vi "MQTT_SubAck_Send.vi"(8 "error in (no error)":errorcluster, 9 "Granted QoS Levels":T2[](array[typedef]), 10 "Message ID":u16=10 format="%x", 11 "SSL_Connection":T1) -> (0 "error out":errorcluster, 2 "Suback Message":u8[](array[numeric]) format="%x", 3 "SSL_Connection":T1)   [LabVIEW 2018, in "AWS_IoT.lvlib"]
uses:
  AWS_IoT.lvlib
  Controls/QoS.ctl
  Controls/SSL_Connection.ctl
  Controls/MessageType.ctl
  Controls/Retain_Flag.ctl
  Controls/DUP_Flag.ctl
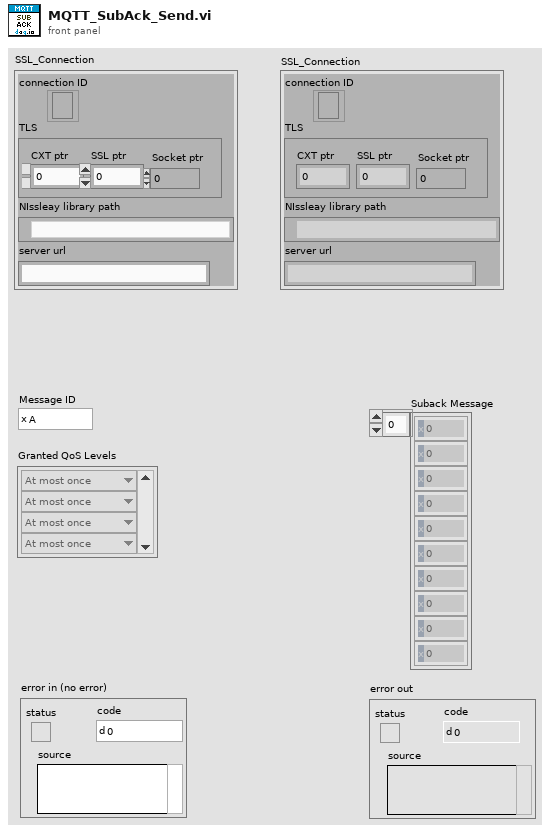
[diagram p1: front panel]
types:
  T1 = typedef "AWS_IoT.lvlib/SSL_Connection.ctl" = cluster{"connection ID":refnum<k5>, "TLS":cluster{"CXT ptr":i32, "SSL ptr":i32, "Socket ptr":i32}, "NIssleay library path":path, "server url":string}
  T2 = typedef "AWS_IoT.lvlib/QoS.ctl" = enum8{"At most once", "At least once", "Exactly once", "Reserved"}
  T3 = typedef "AWS_IoT.lvlib/DUP_Flag.ctl" = bool
  T4 = typedef "AWS_IoT.lvlib/Retain_Flag.ctl" = bool
  T5 = typedef "AWS_IoT.lvlib/MessageType.ctl" = enum32{"Reserved", "CONNECT", "CONNACK", "PUBLISH", "PUBACK", "PUBREC", "PUBREL", "PUBCOMP", "SUBSCRIBE", "SUBACK", "UNSUBSCRIBE", "UNSUBACK", "PINGREQ", "PINGRESP", "DISCONNECT", "Reserved2"}
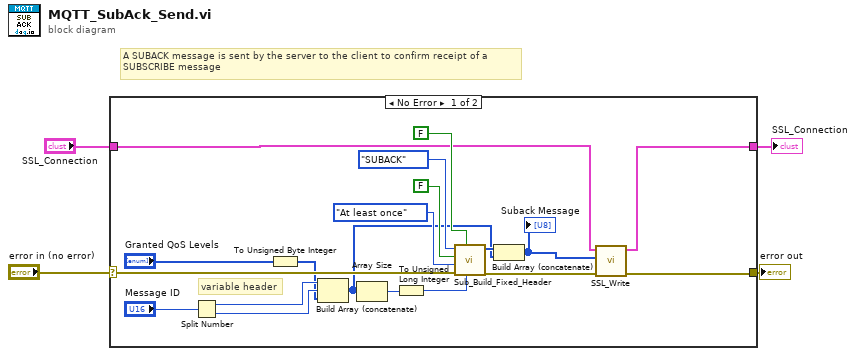
[diagram p0: block diagram]
diagram:
  # "A SUBACK message is sent by the server to the client to confirm receipt of a\nSUBSCRIBE message"
  n1 = case shown="No Error" "error in (no error)" {
    selector: "error in (no error)" -> [w15 w25]
    tunnel: [w9 w25] -> w3
    tunnel: "SSL_Connection" -> [w6 w24]
    tunnel: [w5 w24] -> w1
    frame No Error {
      # "variable header"
      n2 = Split Number(x="Message ID") -> (hi(x)=w21:u8, lo(x)=w20:u8)
      n3 = To Unsigned Byte Integer(number="Granted QoS Levels") -> (unsigned 8bit integer=w10:u8[])
      n4 = Build Array (concatenate)(w21, w20, w10) -> (w14:u8[])
      n5 = Array Size(array=w14) -> (size(s)=w13:i32)
      n6 = To Unsigned Long Integer(number=w13) -> (unsigned 32bit integer=w12:u32)
      n7 = call "Sub_Build_Fixed_Header.vi"("Remaining Length"=w12, "Retain"=T4 FALSE, "error in (no error)"=w15, "QoS"=QoS."At least once", "DUP"=T3 FALSE, "MessageType"=MessageType."SUBACK") -> ("error out"=w8:errorcluster, "Fixed Header"=w22:u8[])  [unwired: 4 in]
      n8 = Build Array (concatenate)(w22, w14) -> (w7:u8[])
      "Suback Message" <- w7
      n9 = call "SSL_Write.vi"("error in (no error)"=w8, "data in"=w7, "SSL_Connection"=w6) -> ("error out"=w9:errorcluster, "SSL_Connection"=w5:T1)  [unwired: 7 in]
    }
    frame Error {
    }
  }
  "error out" <- w3
  "SSL_Connection" <- w1
